vi "Another method by miss.vi"() -> ()   [LabVIEW 2021]
panel:
  out "?":bool
  in  "?":bool
  in  "Password:":string
  in  "Username:":string
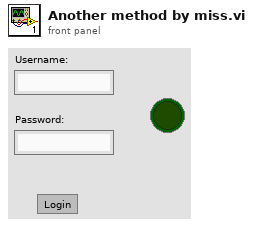
[diagram p1: front panel]
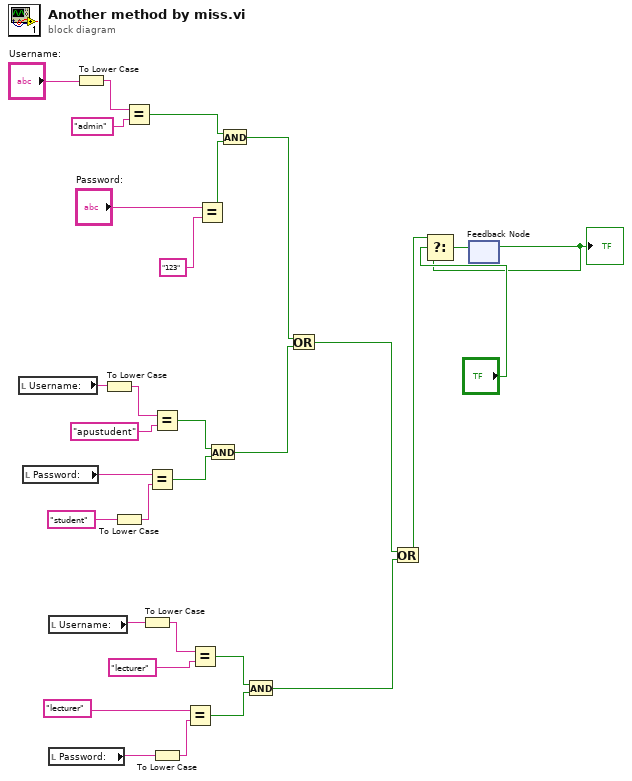
[diagram p0: block diagram]
diagram:
  n1 = local read "Username:"() -> (w21:string)
  n2 = local read "Password:"() -> (w22:string)
  n3 = local read "Username:"() -> (w8:string)
  n4 = local read "Password:"() -> (w7:string)
  n5 = To Lower Case(string="Username:") -> (all lower case string=w30:string)
  n6 = To Lower Case(string=w21) -> (all lower case string=w24:string)
  n7 = To Lower Case(string="student") -> (all lower case string=w20:string)
  n8 = Equal?(x=w30, y="admin") -> (x = y?=w26:bool)
  n9 = To Lower Case(string=w8) -> (all lower case string=w13:string)
  n10 = Equal?(x=w22, y=w20) -> (x = y?=w16:bool)
  n11 = Equal?(x=w24, y="apustudent") -> (x = y?=w17:bool)
  n12 = To Lower Case(string=w7) -> (all lower case string=w11:string)
  n13 = Equal?(x="lecturer", y=w11) -> (x = y?=w9:bool)
  n14 = Equal?(x=w13, y="lecturer") -> (x = y?=w10:bool)
  n15 = Equal?(x="Password:", y="123") -> (x = y?=w25:bool)
  n16 = And(x=w17, y=w16) -> (x .and. y?=w15:bool)
  n17 = And(x=w26, y=w25) -> (x .and. y?=w18:bool)
  n18 = And(x=w10, y=w9) -> (x .and. y?=w4:bool)
  n19 = Or(x=w18, y=w15) -> (x .or. y?=w5:bool)
  n20 = Or(x=w5, y=w4) -> (x .or. y?=w3:bool)
  n21 = feedback #1() -> (w1:bool)  [unwired: 1 in]
  "?" <- w1
  n22 = Select(t=w3, s="?", f=w1) -> (s? t:f=w2:bool)
  n23 = feedback-in #1(w2) -> ()
